vi "Mark10 Speed Calc.vi"(8 "Home to Surface":dbl=2.0 format="%#_13g", 9 "Live Position":dbl step=0.1, 10 "H2S Speed":dbl[](array[numeric]), 11 "H2S %":dbl[](array[numeric])) -> (3 "Speed Output":dbl)   [LabVIEW 2015]
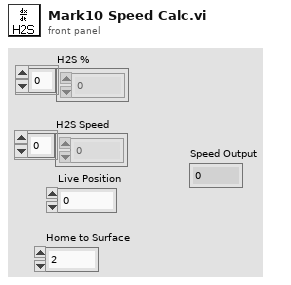
[diagram p1: front panel]
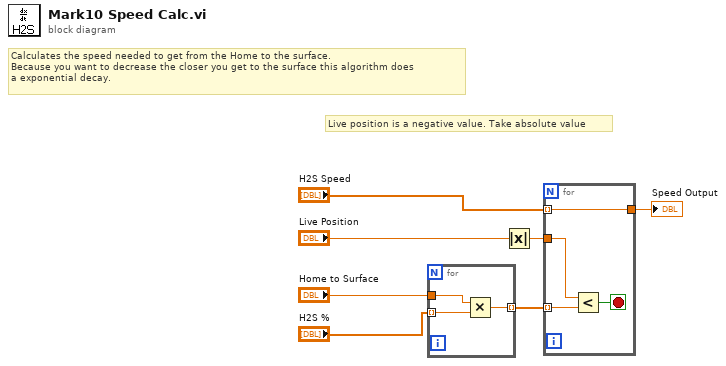
[diagram p0: block diagram]
diagram:
  # "Live position is a negative value. Take absolute value"
  # "Calculates the speed needed to get from the Home to the surface. \nBecause you want to decrease the closer you get to the surface this algorithm does \na exponential decay."
  n1 = for {
    tunnel: "Home to Surface" -> [w10]
    tunnel: "H2S %" -> [w9] mode=indexing
    tunnel: [w8] -> w4 mode=indexing
    n2 = Multiply(x=w10, y=w9) -> (x*y=w8:dbl)
  }
  n3 = Absolute Value(x="Live Position") -> (abs(x)=w5:dbl)
  n4 = for {
    tunnel: w4 -> [w11] mode=indexing
    tunnel: w5 -> [w14]
    tunnel: "H2S Speed" -> [w13] mode=indexing
    tunnel: [w13] -> w7
    stop <- w12 stop-if-true
    n5 = Less?(x=w14, y=w11) -> (x < y?=w12:bool)
  }
  "Speed Output" <- w7
